vi "Close.vi"(8 "error in (no error)":errorcluster, 11 "SQLiteLogHandle in":refnum<class "SQLiteLogHandle.lvclass">) -> (0 "error out":errorcluster)   [LabVIEW 2024, in "SQLiteLogHandle.lvclass"]
uses:
  SQLiteLogHandle.lvclass
  SQLiteLogHandle.lvclass/SQLiteLogHandle.ctl
  <vilib>/drjdpowell/SQLite Library/SQL Statement/SQL Statement.lvclass
  <vilib>/drjdpowell/SQLite Library/SQL Connection/Connection.lvclass
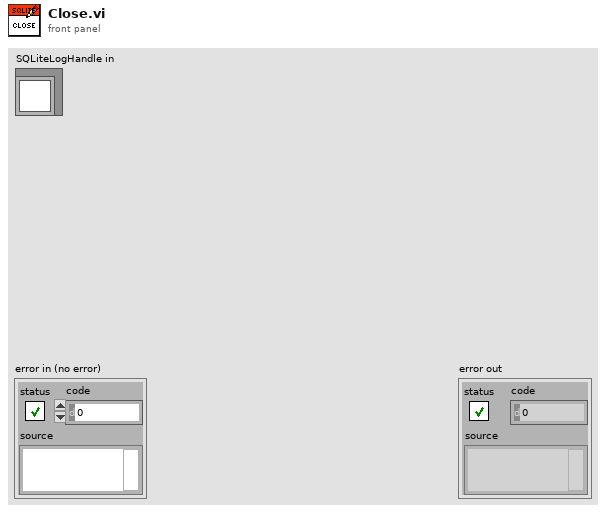
[diagram p1: front panel]
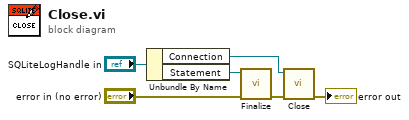
[diagram p0: block diagram]
diagram:
  n1 = Unbundle By Name("SQLiteLogHandle in") -> ("Connection"=w3:refnum<class "Connection.lvclass">, "Statement"=w5:refnum<class "SQL Statement.lvclass">)
  n2 = call <vilib>:"Finalize.vi"("error in (no error)"="error in (no error)", "SQL Statement in"=w5) -> ("error out"=w2:errorcluster)  [unwired: 9 in]
  n3 = call-dynamic "Close.vi"("error in (no error)"=w2, "SQLite Connection in"=w3) -> ("error out"=→"error out":errorcluster)  [unwired: 9 in]
